vi "Write.vi"(1 "Location of DAQ":string, 2 "Temperature from DAQ":dbl=29.983730243560316) -> ()   [LabVIEW 2023]
uses:
  <vilib>/OPCUA/controls/NodeId.ctl
  <vilib>/OPCUA/controls/Write Status.ctl
  <vilib>/OPCUA/client/Multiple Write Double.vi
  <vilib>/OPCUA/client/Multiple Write String.vi
  <vilib>/OPCUA/NI OPC UA Client.lvlib
panel:
  in  "Location Item Path":string="ns=2;s=Location.Location"
  in  "Data Item Path":string="ns=2;s=Data.Temperature"
  in  "Server Endpoint URL":string="opc.tcp://Beist:49580"
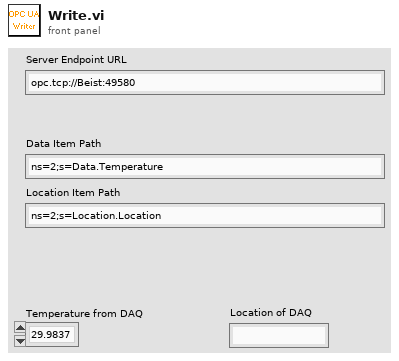
[diagram p1: front panel]
types:
  T1 = typedef "NodeId.ctl" = string
  T2 = typedef "Write Status.ctl" = u32
  T3 = cluster{"node ID":T1, "value":string, "timestamp (current time)":timestamp, "node status":T2}
  T4 = cluster{"node ID":T1, "value":dbl, "timestamp (current time)":timestamp, "node status":T2}
  T5 = cluster{"message mode":enum16{"None", "Sign", "Sign and Encrypt"}, "security":enum16{"Basic256", "Basic128Rsa15"}}
  T6 = cluster{"node ID":T1, "value":dbl, "timestamp (current time)":timestamp, "node status":T2}[]
  T7 = typedef "OPC UA Client Refnum.ctl" = refnum<k21>
  T8 = cluster{"node ID":T1, "value":string, "timestamp (current time)":timestamp, "node status":T2}[]
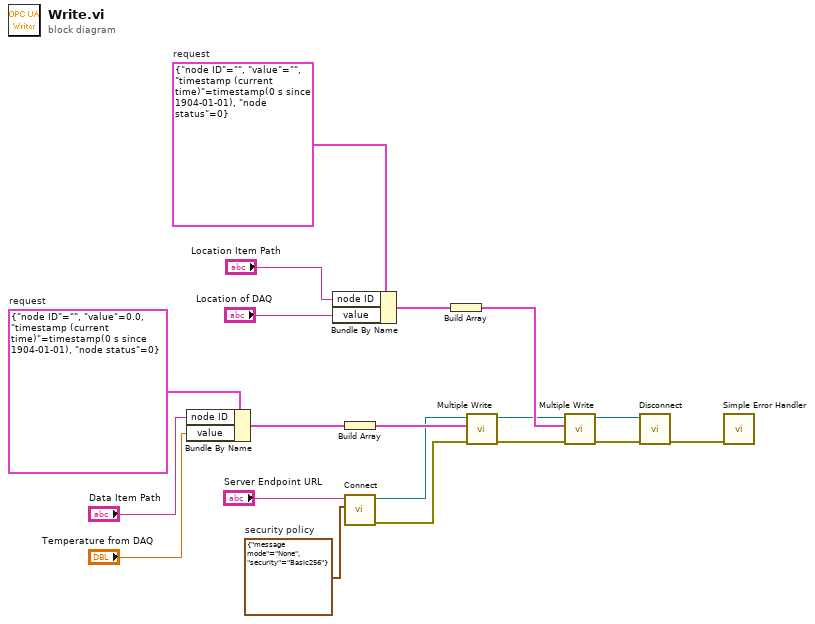
[diagram p0: block diagram]
diagram:
  w9 = T3 {"node ID"="", "value"="", "timestamp (current time)"=timestamp(0 s since 1904-01-01), "node status"=0}  # request
  w12 = T4 {"node ID"="", "value"=0.0, "timestamp (current time)"=timestamp(0 s since 1904-01-01), "node status"=0}  # request
  w19 = T5 {"message mode"=enum."None", "security"=enum."Basic256"}  # security policy
  n1 = Bundle By Name "Bundle By Name"(cluster=w12, "node ID"="Data Item Path", "value"="Temperature from DAQ") -> (w14:T4)
  n2 = Bundle By Name "Bundle By Name"(cluster=w9, "node ID"="Location Item Path", "value"="Location of DAQ") -> (w8:T3)
  n3 = Build Array "Build Array"(w14) -> (w15:T6)
  n4 = call <vilib>:"Connect.vi"("security policy"=w19, "server endpoint URL"="Server Endpoint URL") -> ("error out"=w11:errorcluster, "OPC UA client refnum out"=w10:T7)  [unwired: 7 in, 1 out]
  n5 = Build Array "Build Array"(w8) -> (w5:T8)
  n6 = call-poly <vilib>:"Multiple Write.vi"("error in (no error)"=w11, "requests"=w15, "OPC UA client refnum in"=w10) -> ("error out"=w3:errorcluster, "OPC UA client refnum out"=w4:T7)  [unwired: 5 in, 2 out]
  n7 = call-poly <vilib>:"Multiple Write.vi"("error in (no error)"=w3, "requests"=w5, "OPC UA client refnum in"=w4) -> ("error out"=w2:errorcluster, "OPC UA client refnum out"=w1:T7)  [unwired: 5 in, 2 out]
  n8 = call <vilib>:"Disconnect.vi"("error in (no error)"=w2, "OPC UA client refnum in"=w1) -> ("error out"=w18:errorcluster)  [unwired: 9 in]
  n9 = call <vilib>:"Simple Error Handler.vi"("error in (no error)"=w18) -> ()  [unwired: 4 in, 5 out]
